vi "RT Stream Server.vi"(11 "reader url":string="//192.168.1.125/StatusReader") -> ()   [LabVIEW 2015]
uses:
  Controls/RT Streamer State.ctl
  Controls/RT Streamer Queue element.ctl
  Controls/Generic instruction typedef.ctl
  Controls/LP Status typedef.ctl
  Controls/Log Thread Name.ctl
  <vilib>/dex/Flush And Wait Empty Condition.ctl
  LP Globals.vi
panel:
  out "RT Stream State":T1
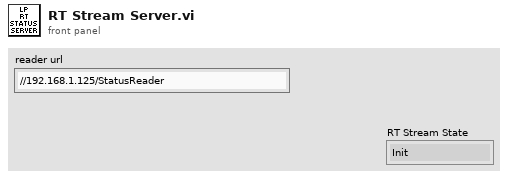
[diagram p1: front panel]
types:
  T1 = typedef "RT Streamer State.ctl" = enum16{"Init", "Idle", "Stream", "Listen", "SetRefrashRate", "SendCmdAck", "SendCmdDone", "SendSysState", "StartRecord", "Error"}
  T2 = typedef "RT Streamer Queue element.ctl" = cluster{"CMD":T1, "Data":variant}
  T3 = cluster{"RefreshRate":i32, "StreamRef":refnum<k21>}
  T4 = typedef "Generic instruction typedef.ctl" = cluster{"CMD":string, "Data":variant}
  T5 = typedef "LP Status typedef.ctl" = cluster{"FrameRate":dbl, "AlgoTime":dbl, "FrameRec":u16}
  T6 = typedef "Log Thread Name.ctl" = enum16{"Motor R", "Generic", "Motor P", "Motor Y", "StreamClient", "Stream Server", "Sequencer"}
  T7 = typedef "Flush And Wait Empty Condition.ctl" = u8
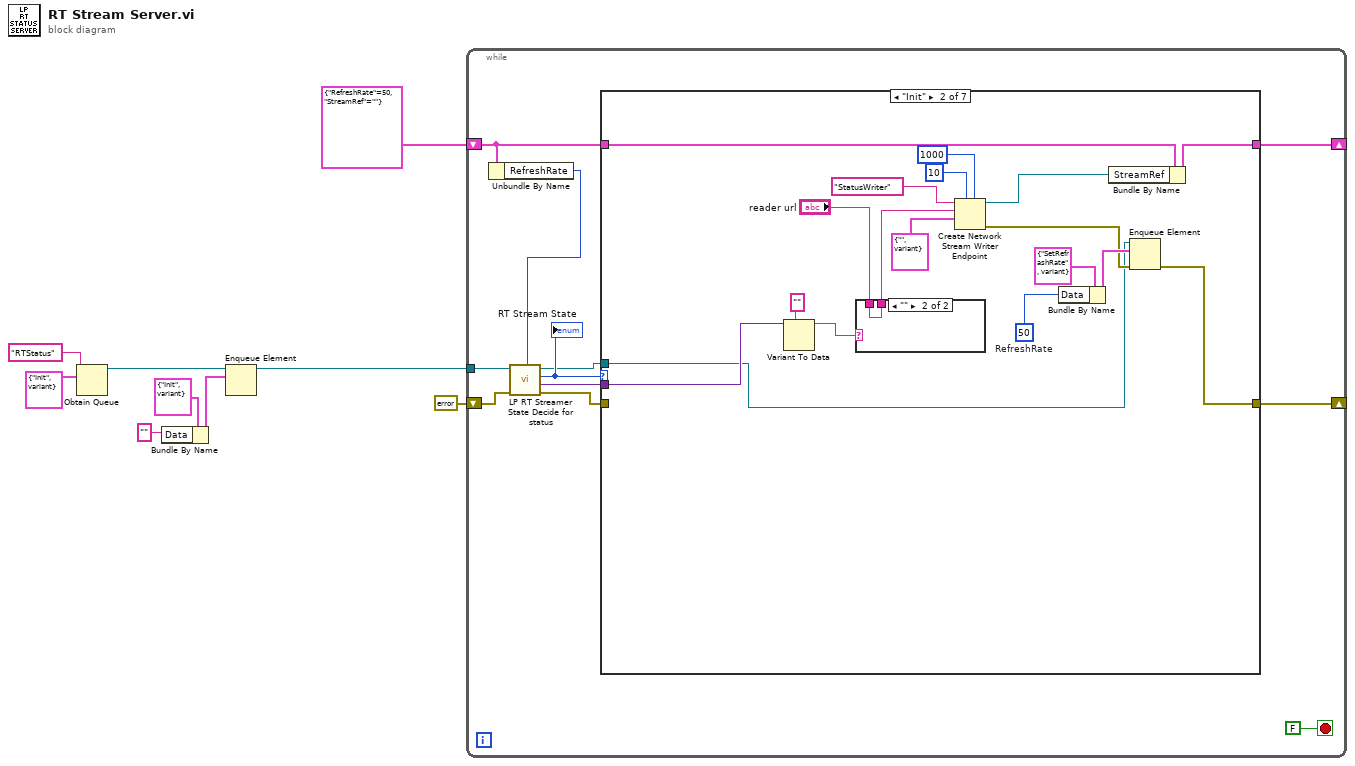
[diagram p0: block diagram]
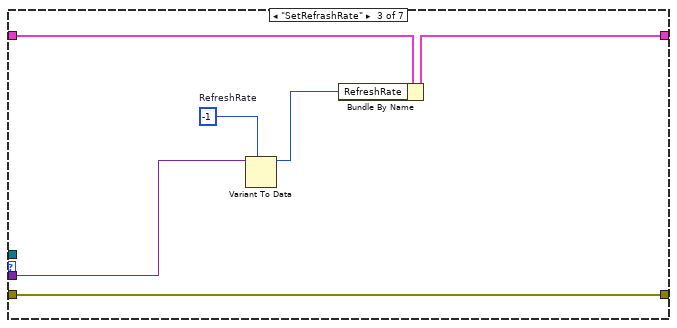
[diagram p4: hidden frame]
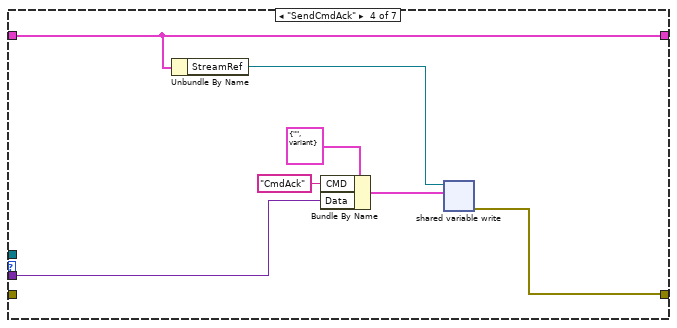
[diagram p5: hidden frame]
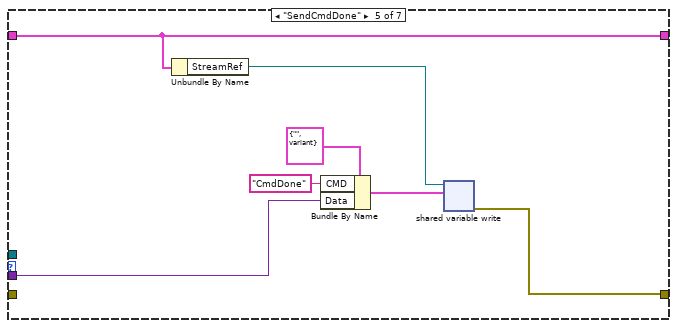
[diagram p6: hidden frame]
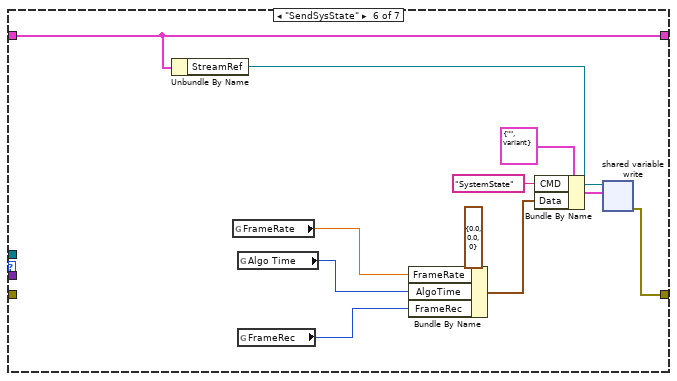
[diagram p7: hidden frame]
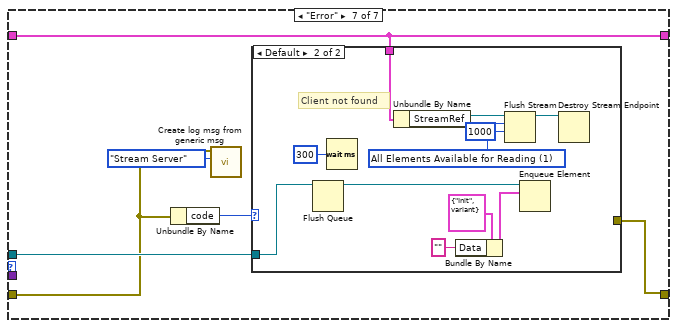
[diagram p8: hidden frame]
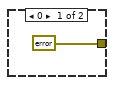
[diagram p9: hidden frame]
diagram:
  n1 = Obtain Queue(name (unnamed)="RTStatus", element data type=T2 {"CMD"=enum."Init", "Data"=variant}) -> (queue out=w6:refnum<queue>)  [unwired: 3 in, 2 out]
  n2 = Bundle By Name(cluster=T2 {"CMD"=enum."Init", "Data"=variant} ("element"), "Data"="") -> (w4:T2)
  n3 = Enqueue Element(queue=w6, element=w4) -> (queue out=w1:refnum<queue>)  [unwired: 2 in, 2 out]
  n4 = while {
    shift-right: [w18] -> _
    shift-left: T3 {"RefreshRate"=50, "StreamRef"=""} -> [w16]
    shift-right: [w20] -> _
    shift-left: errorcluster {"status"=FALSE, "code"=0, "source"=""} ("error constant") -> [w12]
    tunnel: w1 -> [w19]
    stop <- FALSE stop-if-true
    n5 = Unbundle By Name(w16) -> ("RefreshRate"=w15:i32)
    n6 = call "LP RT Streamer State Decide for status.vi"("error in (no error)"=w12, "RefreshRate"=w15, "Queue in"=w19) -> ("error out"=w11:errorcluster, "Data"=w10:variant, "CMD"=w14:T1, "queue out"=w13:refnum<queue>)  [unwired: 5 in]
    "RT Stream State" <- w14
    n7 = case shown="\"Init\"" w14 {
      tunnel: [w21 w25 w44 w49 w56 w68 w78] -> w20
      tunnel: w16 -> [w22 w39 w46 w55 w62 w73 w76]
      tunnel: [w22 w38 w45 w55 w62 w73 w76] -> w18
      tunnel: w10 -> [_ w37 w48 w50 w57 _ _]
      tunnel: w11 -> [w21 _ w44 _ _ _ w75]
      tunnel: w13 -> [_ w24 _ _ _ _ w77]
      frame "Idle", Default {
      }
      frame "Init" {
        w29 = 50  # RefreshRate
        n8 = Variant To Data(type="", Variant=w37) -> (data=w35:string)  [unwired: 1 in, 1 out]
        n9 = case shown="\"\"" w35 {
          selector: w35 -> [w41 _]
          tunnel: "reader url" -> [_ w42]
          tunnel: [w41 w42] -> w23
          frame Default {
          }
          frame "" {
          }
        }
        n10 = Create Network Stream Writer Endpoint(5:1000 ("timeout in ms (-1)"), 7:10 ("writer buffer size"), 9:T4 {"CMD"="", "Data"=variant}, 10:w23, 11:"StatusWriter" ("writer name")) -> (0:w26:errorcluster, 3:w30:refnum<k21>)  [unwired: 2 in]
        n11 = Bundle By Name(cluster=T2 {"CMD"=enum."SetRefrashRate", "Data"=variant} ("element"), "Data"=w29) -> (w28:T2)
        n12 = Bundle By Name(cluster=w39, "StreamRef"=w30) -> (w38:T3)
        n13 = Enqueue Element(queue=w24, element=w28, error in (no error)=w26) -> (error out=w25:errorcluster)  [unwired: 1 in, 2 out]
      }
      frame "SetRefrashRate" {
        w47 = -1  # RefreshRate
        n14 = Variant To Data(type=w47, Variant=w48) -> (data=w43:i32)  [unwired: 1 in, 1 out]
        n15 = Bundle By Name(cluster=w46, "RefreshRate"=w43) -> (w45:T3)
      }
      frame "SendCmdAck" {
        n16 = Unbundle By Name(w55) -> ("StreamRef"=w51:refnum<k21>)
        n17 = Bundle By Name(cluster=T4 {"CMD"="", "Data"=variant}, "CMD"="CmdAck", "Data"=w50) -> (w52:T4)
        n18 = shared-variable-write(w51, w52) -> (w49:errorcluster)  [unwired: 2 in, 2 out]
      }
      frame "SendCmdDone" {
        n19 = Unbundle By Name(w62) -> ("StreamRef"=w58:refnum<k21>)
        n20 = Bundle By Name(cluster=T4 {"CMD"="", "Data"=variant}, "CMD"="CmdDone", "Data"=w57) -> (w59:T4)
        n21 = shared-variable-write(w58, w59) -> (w56:errorcluster)  [unwired: 2 in, 2 out]
      }
      frame "SendSysState" {
        n22 = Unbundle By Name(w73) -> ("StreamRef"=w69:refnum<k21>)
        n23 = global read "LP Globals.vi" "FrameRate"() -> (w65:dbl)
        n24 = global read "LP Globals.vi" "Algo Time"() -> (w64:u32)
        n25 = global read "LP Globals.vi" "FrameRec"() -> (w63:u16)
        n26 = Bundle By Name(cluster=T5 {"FrameRate"=0.0, "AlgoTime"=0.0, "FrameRec"=0} ("LP Status"), "FrameRate"=w65, "AlgoTime"=w64, "FrameRec"=w63) -> (w66:T5)
        n27 = Bundle By Name(cluster=T4 {"CMD"="", "Data"=variant}, "CMD"="SystemState", "Data"=w66) -> (w70:T4)
        n28 = shared-variable-write(w69, w70) -> (w68:errorcluster)  [unwired: 2 in, 2 out]
      }
      frame "Error" {
        n29 = Unbundle By Name(w75) -> ("code"=w79:i32)
        n30 = call "Create log msg from generic msg.vi"("Thread"=Log_Thread_Name."Stream Server", "variant"=w75) -> ()  [unwired: 10 in]
        n31 = case shown="Default" w79 {
          tunnel: [errorcluster {"status"=FALSE, "code"=0, "source"=""} ("error constant") _] -> w78
          tunnel: w77 -> [_ w87]
          tunnel: w76 -> [_ w85]
          frame 0 {
          }
          frame Default {
            w84 = T7 1 items=["All Elements Read From Stream", "All Elements Available for Reading"] ("wait condition")
            # "Client not found"
            n32 = Flush Queue(queue=w87) -> (queue out=w86:refnum<queue>)  [unwired: 1 in, 2 out]
            n33 = Wait (ms)(milliseconds to wait=u32 300) -> ()  [unwired: 1 out]
            n34 = Unbundle By Name(w85) -> ("StreamRef"=w81:refnum<k21>)
            n35 = Bundle By Name(cluster=T2 {"CMD"=enum."Init", "Data"=variant} ("element"), "Data"="") -> (w89:T2)
            n36 = Flush Stream(9:1000 ("timeout in ms (-1)"), 10:w84, 11:w81) -> (3:w82:refnum<k21>)  [unwired: 1 in, 2 out]
            n37 = Enqueue Element(queue=w86, element=w89) -> ()  [unwired: 2 in, 3 out]
            n38 = Destroy Stream Endpoint(11:w82) -> ()  [unwired: 1 in, 1 out]
          }
        }
      }
    }
  }
